vi "SendSMTP_Email.vi"(4 "Send as attachment":bool, 5 "message":string="This email was sent to you via labview SMTP email.!", 6 "message (attachment)":string, 7 "subject ([No Subject])":string="<Automatic Email> Do not respond!", 8 "error in (no error)":errorcluster, 10 "file path":path, 11 "Recipient Email Address":string) -> (0 "error out":errorcluster)   [LabVIEW 2018]
panel:
  in  "max iter":i32=10
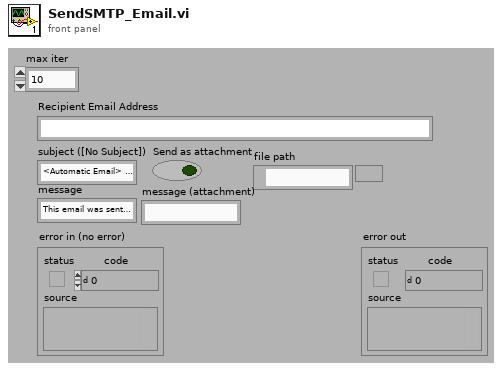
[diagram p1: front panel]
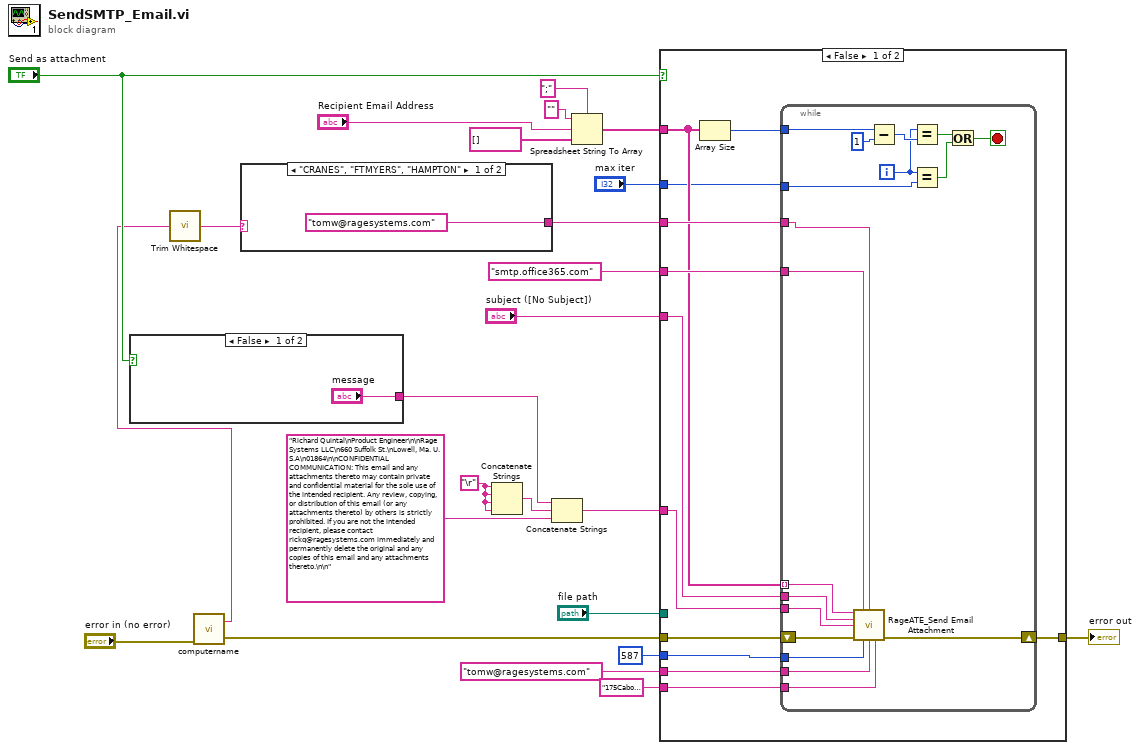
[diagram p0: block diagram]
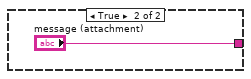
[diagram p2: hidden frame]
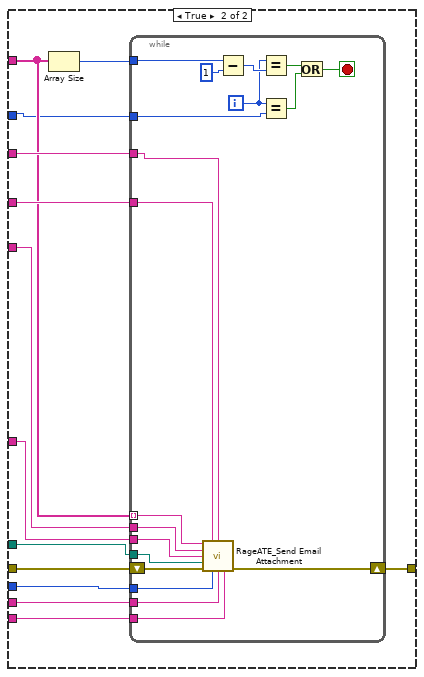
[diagram p3: hidden frame]
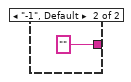
[diagram p4: hidden frame]
diagram:
  w12 = "\r"
  n1 = case shown="False" "Send as attachment" {
    tunnel: ["message" "message (attachment)"] -> w15
    frame False {
    }
    frame True {
    }
  }
  n2 = call "computername.vi"("error in (no error)"="error in (no error)") -> ("error out"=w20:errorcluster, "String/Binary data"=w2:string)  [unwired: 3 in]
  n3 = call <vilib>:"Trim Whitespace.vi"("string"=w2) -> ("trimmed string"=w1:string)  [unwired: 1 in]
  n4 = case shown="\"CRANES\", \"FTMYERS\", \"HAMPTON\"" w1 {
    tunnel: ["tomw@ragesystems.com" ("Mail Server 2") "" ("Mail Server 2")] -> w22
    frame "CRANES", "FTMYERS", "HAMPTON" {
    }
    frame "-1", Default {
    }
  }
  n5 = Concatenate Strings(w12, w12, w12, w12) -> (w13:string)
  n6 = Concatenate Strings(w15, w13, "Richard Quintal\nProduct Engineer\n\nRage Systems LLC\n660 Suffolk St.\nLowell, Ma. U.S.A\n01864\n\nCONFIDENTIAL COMMUNICATION: This email and any attachments thereto may contain private and confidential material for the sole use of the intended recipient. Any review, copying, or distribution of this email (or any attachments thereto) by others is strictly prohibited. If you are not the intended recipient, please contact rickq@ragesystems.com immediately and permanently delete the original and any copies of this email and any attachments thereto.\n\n") -> (w14:string)
  n7 = Spreadsheet String To Array(delimiter (Tab)=";", format string="", spreadsheet string="Recipient Email Address", array type (2D Dbl)=string[] []) -> (array=w6:string[])
  n8 = case shown="False" "Send as attachment" {
    tunnel: "subject ([No Subject])" -> [w40 w71]
    tunnel: w6 -> [w31 w62]
    tunnel: w14 -> [w39 w70]
    tunnel: [w38 w69] -> w23
    tunnel: w22 -> [w37 w68]
    tunnel: w20 -> [w36 w67]
    tunnel: "tomw@ragesystems.com" ("Email Account ID") -> [w34 w65]
    tunnel: "175CabotSt!" ("Email Account Password") -> [w35 w66]
    tunnel: 587 ("Port") -> [w33 w64]
    tunnel: "smtp.office365.com" ("SMTP Outgoing Mail Server") -> [w32 w63]
    tunnel: "file path" -> [_ w59]
    tunnel: "max iter" -> [w29 w60]
    frame False {
      n9 = Array Size(array=w31) -> (size(s)=w30:i32)
      n10 = while {
        tunnel: w40 -> [w58]
        tunnel: w31 -> [w57] mode=indexing
        tunnel: w39 -> [w49]
        tunnel: w37 -> [w55]
        tunnel: w35 -> [w53]
        tunnel: w34 -> [w52]
        tunnel: w33 -> [w51]
        tunnel: w32 -> [w50]
        shift-right: [w56] -> w38
        shift-left: w36 -> [w54]
        tunnel: w30 -> [w45]
        tunnel: w29 -> [w41]
        i -> [w42]
        stop <- w48 stop-if-true
        n11 = call "RageATE_Send Email Attachment.vi"("To: (email@site.com)"=w57, "SMTP Outgoing Mail Server"=w50, "From: (email@site.com)"=w55, "Subject:"=w58, "Body:"=w49, "error in (no error)"=w54, "Port"=w51, "Email Account ID"=w52, "Email Account Password"=w53) -> ("error out"=w56:errorcluster)  [unwired: 6 in]
        n12 = Subtract(x=w45, y=1) -> (x-y=w46:i32)
        n13 = Equal?(x=w42, y=w46) -> (x = y?=w47:bool)
        n14 = Equal?(x=w42, y=w41) -> (x = y?=w43:bool)
        n15 = Or(x=w47, y=w43) -> (x .or. y?=w48:bool)
      }
    }
    frame True {
      n16 = Array Size(array=w62) -> (size(s)=w61:i32)
      n17 = while {
        tunnel: w71 -> [w90]
        tunnel: w62 -> [w89] mode=indexing
        tunnel: w70 -> [w81]
        tunnel: w68 -> [w87]
        tunnel: w66 -> [w85]
        tunnel: w65 -> [w84]
        tunnel: w64 -> [w83]
        tunnel: w63 -> [w82]
        shift-right: [w88] -> w69
        shift-left: w67 -> [w86]
        tunnel: w61 -> [w77]
        tunnel: w60 -> [w73]
        tunnel: w59 -> [w72]
        i -> [w74]
        stop <- w80 stop-if-true
        n18 = call "RageATE_Send Email Attachment.vi"("To: (email@site.com)"=w89, "SMTP Outgoing Mail Server"=w82, "From: (email@site.com)"=w87, "Subject:"=w90, "Body:"=w81, "Attachment Path"=w72, "error in (no error)"=w86, "Port"=w83, "Email Account ID"=w84, "Email Account Password"=w85) -> ("error out"=w88:errorcluster)  [unwired: 5 in]
        n19 = Subtract(x=w77, y=1) -> (x-y=w78:i32)
        n20 = Equal?(x=w74, y=w78) -> (x = y?=w79:bool)
        n21 = Equal?(x=w74, y=w73) -> (x = y?=w75:bool)
        n22 = Or(x=w79, y=w75) -> (x .or. y?=w80:bool)
      }
    }
  }
  "error out" <- w23
